vi "Check Limitation.vi"(10 "Value":dbl format="%.6f", 11 "Limit":cluster{"Max":dbl, "Min":dbl}) -> (1 "Result Out":string, 2 "In Range?":bool, 3 "Color Box":u32(colorbox)=6618880)   [LabVIEW 2015, in "SQLite.lvclass"]
uses:
  SQLite.lvclass
panel:
  out "1: OK; 2: NG":i16
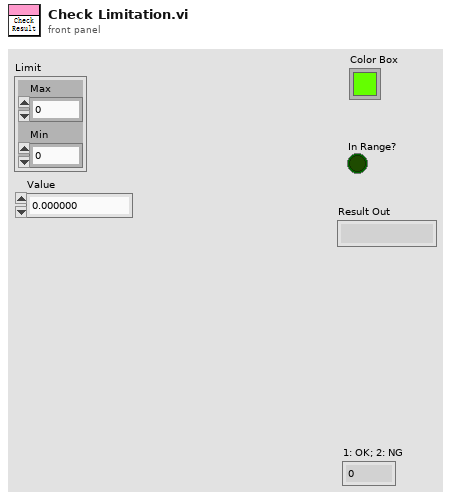
[diagram p1: front panel]
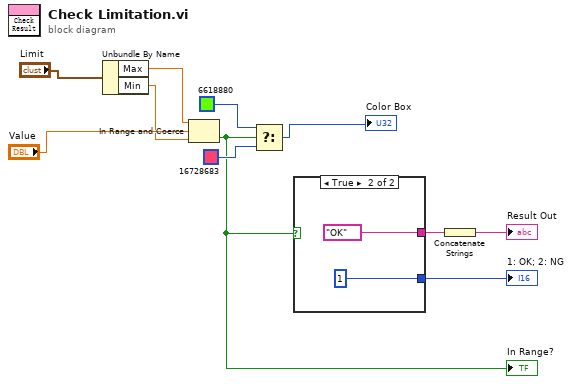
[diagram p0: block diagram]
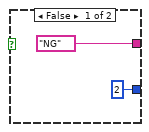
[diagram p2: hidden frame]
diagram:
  n1 = Unbundle By Name("Limit") -> ("Max"=w7:dbl, "Min"=w6:dbl)
  n2 = In Range and Coerce(upper limit=w7, x="Value", lower limit=w6) -> (In Range?=w1:bool)  [unwired: 1 out]
  "In Range?" <- w1
  n3 = Select(t=u32 6618880, s=w1, f=u32 16728683) -> (s? t:f=→"Color Box":u32)
  n4 = case shown="True" w1 {
    tunnel: ["NG" ("Result") "OK" ("Result")] -> w2
    tunnel: [i16 2 ("0, 2") i16 1 ("0, 2")] -> w4
    frame False {
    }
    frame True {
    }
  }
  "1: OK; 2: NG" <- w4
  n5 = Concatenate Strings(w2) -> (→"Result Out":string)
